vi "Get Property Values (String Properties).vi"(1 "data type":string[][](array[string]), 5 "properties":T1[](array[typedef]) {"data type" items=["Unknown"=0, "String"=23, "I32"=3, "I64"=4, "DBL"=10, "Time stamp"=30]; "object type" items=["File", "Channel Group", "Channel"]}, 7 "result references":T4[](array[typedef]), 11 "error in (no error)":errorcluster) -> (6 "property values":string[][](array[string]), 8 "result references out":T4[](array[typedef]), 15 "error out":errorcluster)   [LabVIEW 2020, in "NI_DataFinder.lvlib"]
doc: "Determines from the result references the values of string properties."
uses:
  <vilib>/DataFinder/NI_DataFinder.lvlib
  <vilib>/DataFinder/DataTypes/property.ctl
  <vilib>/DataFinder/DataTypes/object type.ctl
  <vilib>/DataFinder/DataTypes/data type.ctl
  <vilib>/userdefined/DFSearchResult.ctl
  <vilib>/userdefined/NI_DataFinder Controls.lvlib
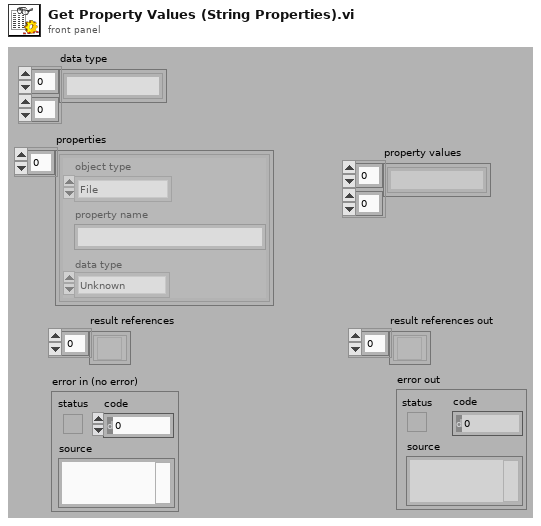
[diagram p1: front panel]
types:
  T1 = typedef "NI_DataFinder.lvlib/property.ctl" = cluster{"object type":T2, "property name":string, "data type":T3}
  T2 = typedef "NI_DataFinder.lvlib/object type.ctl" = u16
  T3 = typedef "NI_DataFinder.lvlib/data type.ctl" = u16
  T4 = typedef "NI_DataFinder Controls.lvlib/DFSearchResult.ctl" = refnum<k20>
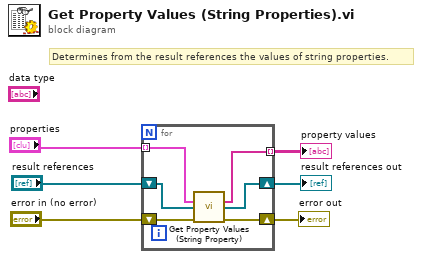
[diagram p0: block diagram]
diagram:
  # "Determines from the result references the values of string properties."
  n1 = for {
    tunnel: "properties" -> [w10] mode=indexing
    tunnel: [w11] -> w5 mode=indexing
    shift-right: [w8] -> w2
    shift-left: "error in (no error)" -> [w12]
    shift-right: [w7] -> w1
    shift-left: "result references" -> [w9]
    n2 = call <vilib>:"Get Property Values (String Property).vi"("property"=w10, "result references"=w9, "error in (no error)"=w12) -> ("property values"=w11:string[], "result references out"=w7:T4[], "error out"=w8:errorcluster)  [unwired: 1 in, 9 out]
  }
  "error out" <- w2
  "result references out" <- w1
  "property values" <- w5
